vi "Read FIeld value.vi"(8 "error in (no error)":errorcluster, 11 "IP Address":string="128.174.165.97") -> (0 "error out":errorcluster, 1 "Z FIeld mT":dbl, 2 "Y Field mT":dbl, 3 "X Field mT":dbl)   [LabVIEW 2024]
panel:
  out "Response String":string
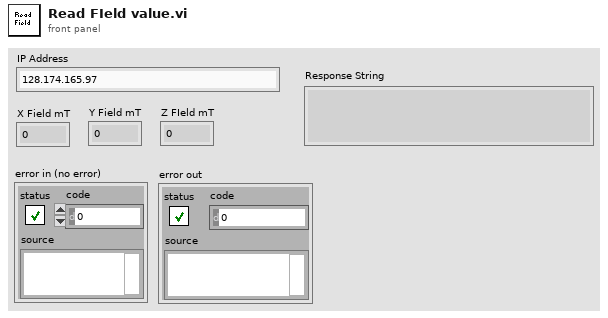
[diagram p1: front panel]
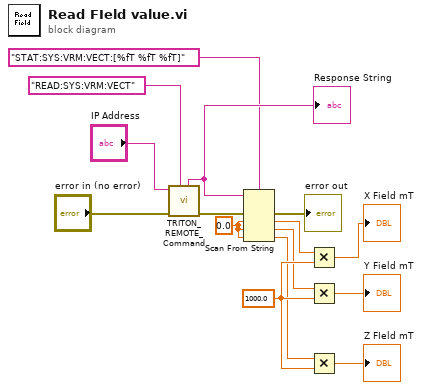
[diagram p0: block diagram]
diagram:
  w7 = 1000.0 ("y")
  w9 = 0.0 ("default value 1")
  n1 = call "TRITON_REMOTE_Command.vi"("Command to send"="READ:SYS:VRM:VECT", "error in (no error)"="error in (no error)", "IP Address"="IP Address") -> ("error out"=w10:errorcluster, "Response String"=w12:string)  [unwired: 6 in, 1 out]
  "Response String" <- w12
  n2 = Scan From String(format string="STAT:SYS:VRM:VECT:[%fT %fT %fT]", input string=w12, error in=w10, default 1=w9, default 2=w9, default 3=w9) -> (error out=→"error out":errorcluster, output 1=w8:dbl, output 2=w6:dbl, output 3=w5:dbl)  [unwired: 1 in, 2 out]
  n3 = Multiply(x=w8, y=w7) -> (x*y=→"X Field mT":dbl)
  n4 = Multiply(x=w6, y=w7) -> (x*y=→"Y Field mT":dbl)
  n5 = Multiply(x=w5, y=w7) -> (x*y=→"Z FIeld mT":dbl)
